vi "UnregisterForMessageSpecificType.vi"(8 "error in (no error)":errorcluster, 9 "Message Enqueuer":refnum<class "Message Enqueuer.lvclass">, 10 "Message":refnum<class "MailBoxMessage.lvclass">, 11 "MailboxManager in":refnum<class "MailboxManager.lvclass">) -> (0 "error out":errorcluster, 3 "MailboxManager out":refnum<class "MailboxManager.lvclass">)   [LabVIEW 2020, in "MailboxManager.lvlib" / "MailboxManager.lvclass"]
uses:
  MailboxManager.lvclass
  MailBoxMessage/MailBoxMessage.lvclass
  <vilib>/ActorFramework/Message Enqueuer/Message Enqueuer.lvclass
  MailboxManager.lvclass/MailboxManager.ctl
  <vilib>/Utility/miscctls.llb/LVMapReplaceAction.ctl
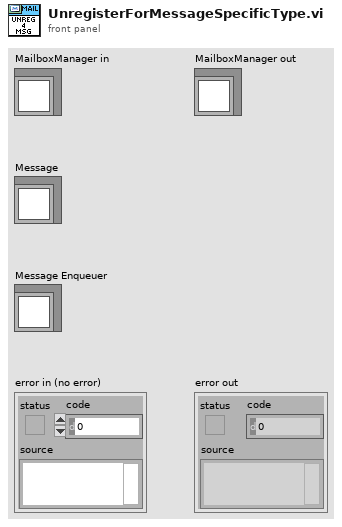
[diagram p1: front panel]
types:
  T1 = typedef "LVMapReplaceAction.ctl" = enum32{"Modify Entry only if found", "Add or Modify Entry", "Delete Entry"}
  T2 = map{refnum<class "MailBoxMessage.lvclass">, refnum<class "Message Enqueuer.lvclass">[]}
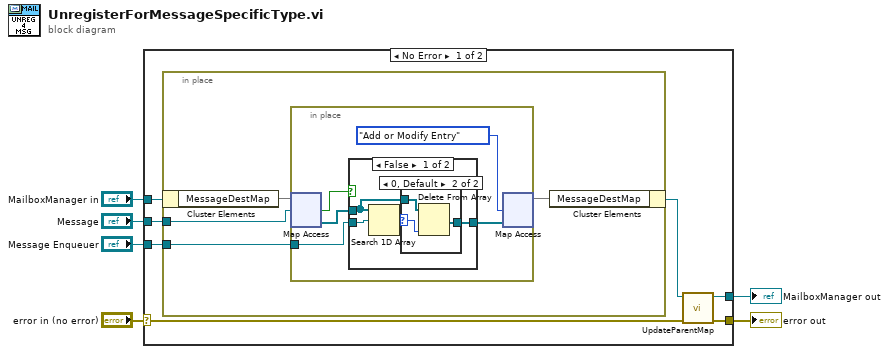
[diagram p0: block diagram]
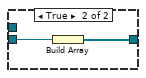
[diagram p3: hidden frame]
diagram:
  n1 = case shown="No Error" "error in (no error)" {
    selector: "error in (no error)" -> [w8 w34]
    tunnel: [w7 w34] -> w5
    tunnel: [w9 w33] -> w3
    tunnel: "MailboxManager in" -> [w13 w33]
    tunnel: "Message Enqueuer" -> [w11 _]
    tunnel: "Message" -> [w12 _]
    frame No Error {
      n2 = in-place {
        in-place-border: w12 -> [w14]
        in-place-border: w11 -> [w16]
        n3 = in-place-cluster #1(w13) -> ("MessageDestMap"=w17:T2)
        n4 = in-place {
          in-place-border: w16 -> [w19]
          n5 = in-place-map #2(w17, w14) -> (w22:refnum<class "Message Enqueuer.lvclass">[], w20:bool)  [unwired: 1 in]
          n6 = case shown="False" w20 {
            tunnel: w22 -> [w24 _]
            tunnel: [w23 w31] -> w21
            tunnel: w19 -> [w26 w32]
            frame False {
              n7 = Search 1D Array(1D array=w24, element=w26) -> (index of element=w25:i32)  [unwired: 1 in]
              n8 = case shown="0, Default" w25 {
                selector: w25 -> [_ w29]
                tunnel: w24 -> [w27 w30]
                tunnel: [w27 w28] -> w23
                frame -1 {
                }
                frame 0, Default {
                  n9 = Delete From Array(array=w30, index=w29) -> (array with subset deleted=w28:refnum<class "Message Enqueuer.lvclass">[])  [unwired: 1 in, 1 out]
                }
              }
            }
            frame True {
              n10 = Build Array(w32) -> (w31:refnum<class "Message Enqueuer.lvclass">[])
            }
          }
          n11 = in-place-map #2(w21, LVMapReplaceAction."Add or Modify Entry" ("action")) -> (w15:T2)  [unwired: 2 out]
        }
        n12 = in-place-cluster #1("MessageDestMap"=w15) -> (w10:refnum<class "MailboxManager.lvclass">)
      }
      n13 = call "UpdateParentMap.vi"("error in (no error)"=w8, "MailboxManager in"=w10) -> ("error out"=w7:errorcluster, "MailboxManager out"=w9:refnum<class "MailboxManager.lvclass">)  [unwired: 8 in]
    }
    frame Error {
    }
  }
  "error out" <- w5
  "MailboxManager out" <- w3
